vi "Read ctl.vi"(8 "error in":errorcluster, 11 "Update TEC PID in":refnum<class "Update TEC PID.lvclass">) -> (0 "error out":errorcluster, 2 "ctl":cluster{"P":dbl, "I":dbl, "D":dbl}, 3 "Update TEC PID out":refnum<class "Update TEC PID.lvclass">)   [LabVIEW 2015, in "Generic TEC.lvlib" / "Update TEC PID.lvclass"]
uses:
  Update TEC PID.lvclass
  Update TEC PID.lvclass/Update TEC PID.ctl
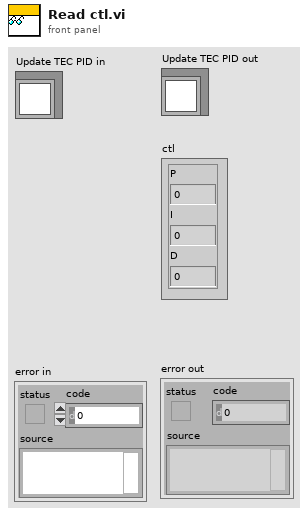
[diagram p1: front panel]
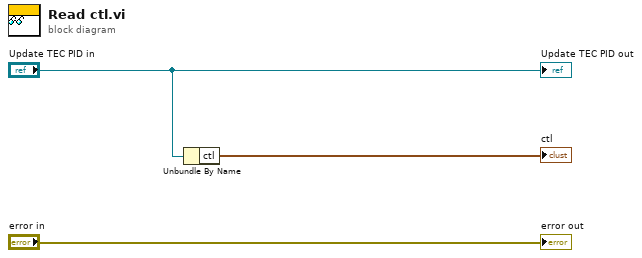
[diagram p0: block diagram]
diagram:
  n1 = Unbundle By Name("Update TEC PID in") -> ("ctl"=→"ctl":cluster{"P":dbl, "I":dbl, "D":dbl})
  "error out" <- "error in"
  "Update TEC PID out" <- "Update TEC PID in"
